vi "Find New Landmarks.vi"(8 "error in (no error)":errorcluster, 10 "SLAM In":T1) -> (0 "error out":errorcluster, 2 "SLAM Out":T1, 3 "New LM's":T3(array[cluster]))   [LabVIEW 2009]
uses:
  Controls/SLAM.ctl
  <vilib>/Analysis/Matrix/Datatypes/RealMatrix.ctl
  <vilib>/Analysis/Matrix/NI_Matrix.lvlib
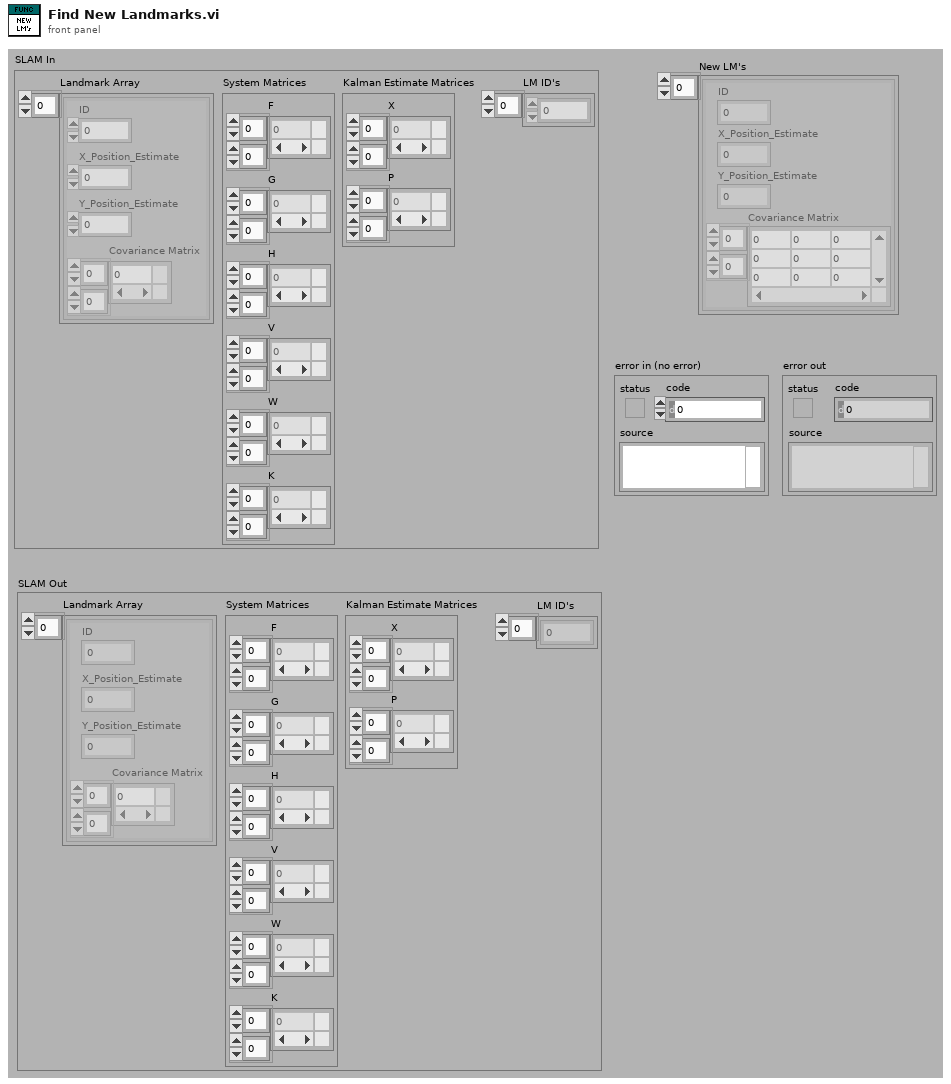
[diagram p1: front panel]
types:
  T1 = typedef "SLAM.ctl" = cluster{"Landmark Array":cluster{"ID":dbl, "X_Position_Estimate":dbl, "Y_Position_Estimate":dbl, "Covariance Matrix":T2}[], "System Matrices":cluster{"F":T2, "G":T2, "H":T2, "V":T2, "W":T2, "K":T2}, "Kalman Estimate Matrices":cluster{"X":T2, "P":T2}, "LM ID's":dbl[]}
  T2 = typedef "NI_Matrix.lvlib/RealMatrix.ctl" = dbl[][]
  T3 = cluster{"ID":dbl, "X_Position_Estimate":dbl, "Y_Position_Estimate":dbl, "Covariance Matrix":T2}[]
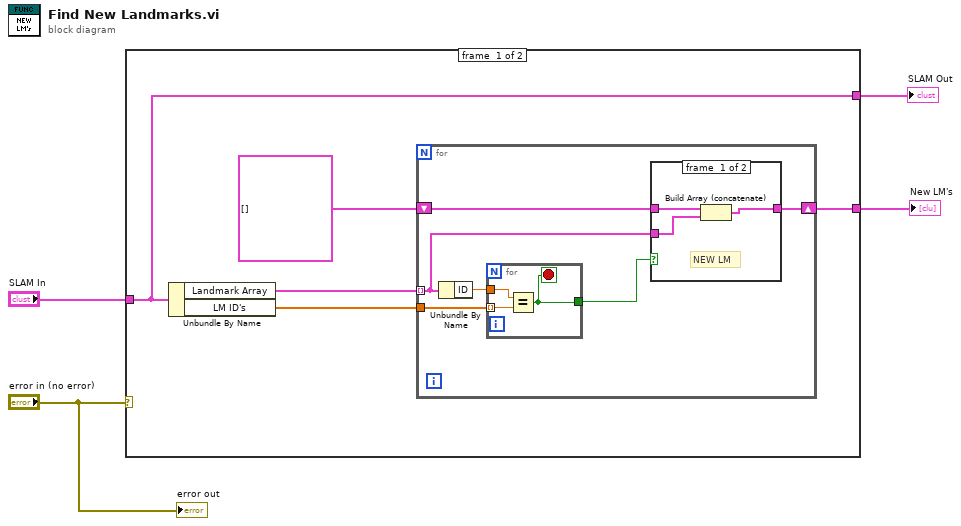
[diagram p0: block diagram]
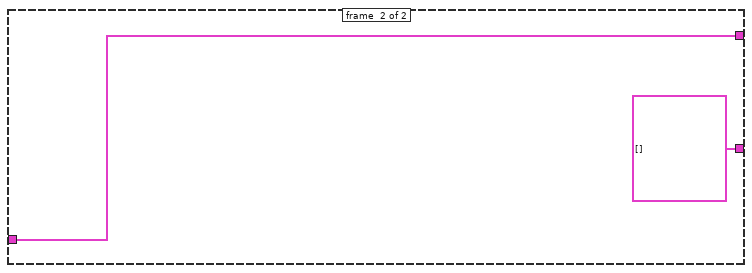
[diagram p3: hidden frame]
diagram:
  n1 = case shown="No Error" "error in (no error)" {
    tunnel: "SLAM In" -> [w5 w23]
    tunnel: [w6 T3 [] ("Landmark Array")] -> w3
    tunnel: [w5 w23] -> w1
    frame #0 {
      n2 = Unbundle By Name(w5) -> ("Landmark Array"=w9:T3, "LM ID's"=w8:dbl[])
      n3 = for {
        tunnel: w9 -> [w11] mode=indexing
        tunnel: w8 -> [w14]
        shift-right: [w10] -> w6
        shift-left: T3 [] ("Landmark Array") -> [w12]
        n4 = Unbundle By Name(w11) -> ("ID"=w15:dbl)
        n5 = for {
          tunnel: w15 -> [w22]
          tunnel: w14 -> [w21] mode=indexing
          tunnel: [w20] -> w13
          stop <- w20 stop-if-true
          n6 = Equal?(x=w22, y=w21) -> (x = y?=w20:bool)
        }
        n7 = case shown="False" w13 {
          tunnel: w12 -> [w18 w19]
          tunnel: [w17 w19] -> w10
          tunnel: w11 -> [w16 _]
          frame #0 {
            # "NEW LM"
            n8 = Build Array (concatenate)(w18, w16) -> (w17:T3)
          }
          frame #1 {
            # "OLD LM"
          }
        }
      }
    }
    frame #1 {
    }
  }
  "New LM's" <- w3
  "SLAM Out" <- w1
  "error out" <- "error in (no error)"
